vi "VI Tree.vi"   [LabVIEW 2015, in "Keysight U1252.lvlib"]
doc: "This is the instrument driver for the <INSTRUMENT NAME>. The VI Tree displays all the user-callable VIs of the instrument driver in an organized table."
uses:
  <instrlib>/Keysight U1252/Keysight U1252.lvlib
  <instrlib>/Keysight U1252/Public/Configure/Low Level/AC Voltage Configuration.vi
panel:
  # "(c) 2014 <Enter Company Name Here>.  ALL RIGHTS RESERVED."
  # "SEE DIAGRAM\nFOR VI TREE."
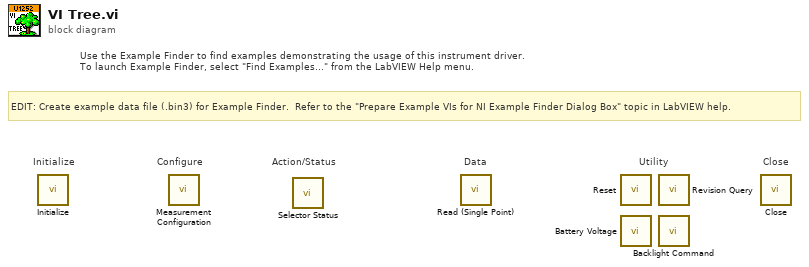
[diagram p0: block diagram]
diagram:
  # "Action/Status"
  # "EDIT: Create example data file (.bin3) for Example Finder.  Refer to the \"Prepare Example VIs for NI Example Finder Dialog Box\" topic in LabVIEW help."
  # "Use the Example Finder to find examples demonstrating the usage of this instrument driver.\nTo launch Example Finder, select \"Find Examples...\" from the LabVIEW Help menu."
  # "Configure"
  # "Utility"
  # "Data"
  # "Close"
  # "Initialize"
  n1 = call <instrlib>:"Initialize.vi"() -> ()  [unwired: 10 in, 2 out]
  n2 = call-poly <instrlib>:"Measurement Configuration.vi"() -> ()  [unwired: 10 in, 2 out]
  n3 = call <instrlib>:"Selector Status.vi"() -> ()  [unwired: 9 in, 3 out]
  n4 = call <instrlib>:"Read (Single Point).vi"() -> ()  [unwired: 9 in, 3 out]
  n5 = call <instrlib>:"Reset.vi"() -> ()  [unwired: 10 in, 2 out]
  n6 = call <instrlib>:"Battery Voltage.vi"() -> ()  [unwired: 9 in, 3 out]
  n7 = call <instrlib>:"Revision Query.vi"() -> ()  [unwired: 6 in, 6 out]
  n8 = call <instrlib>:"Backlight Command.vi"() -> ()  [unwired: 10 in, 2 out]
  n9 = call <instrlib>:"Close.vi"() -> ()  [unwired: 11 in, 1 out]
